vi "ResetDAQmxDevice.vi"(5 "Device":string) -> (0 "error out":errorcluster)   [LabVIEW 2012]
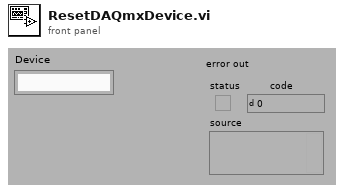
[diagram p1: front panel]
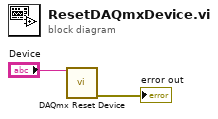
[diagram p0: block diagram]
diagram:
  n1 = call <vilib>:"DAQmx Reset Device.vi"("device in"="Device") -> ("error out"=→"error out":errorcluster)  [unwired: 14 in]
